vi "Enable Disable Input.vi"(8 "Error In":errorcluster, 10 "Disabled":T1(ring)=enum."Disabled", 11 "Input Refs":refnum<vi>[](array[refnum])) -> (0 "error out":errorcluster)   [LabVIEW 2025]
doc: "Enable and disable controls and indicators by reference."
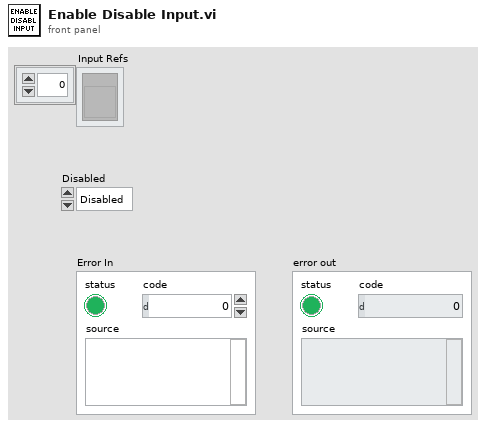
[diagram p1: front panel]
types:
  T1 = enum8{"Enabled", "Disabled", "Disabled and Grayed Out"}
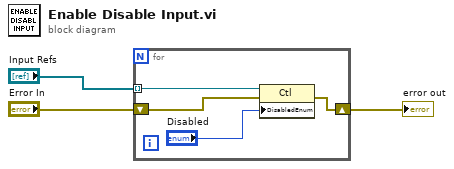
[diagram p0: block diagram]
diagram:
  n1 = for {
    tunnel: "Input Refs" -> [w7] mode=indexing
    shift-right: [w5] -> w2
    shift-left: "Error In" -> [w4]
    n2 = property on="Property Node" class="Ctl"(reference=w7, error in=w4, "DisabledEnum"="Disabled") -> (error out=w5:errorcluster)  [unwired: 1 out]
  }
  "error out" <- w2
